vi "Start Stream.vi"(8 "error in (no error)":errorcluster, 10 "Camera Settings":T1={"Exposure Time (ms)"=100.0, "Binning"=enum."2x2", "Scan Mode"=0, "Frames to Acquire"=1000.0, "Pixel Correction"=FALSE, "Frames to Skip"=0, "File Path"=path "", "Duty cycle"=0.0, "ALEX"=FALSE, "Shutter Enable"=[], "Timelapse Interval (s)"=0, "fluidics trigger frame"=0} {"Timelapse Interval (s)" max=60000 step=1; "Exposure Time (ms)" min=1.0 max=10000.0 step=1.0}, 11 "Orca-Flash 4.0 V2 in":refnum<class "Hamamatsu Camera.lvclass">) -> (0 "error out":errorcluster, 3 "Orca-Flash 4.0 V2 out":refnum<class "Hamamatsu Camera.lvclass">)   [LabVIEW 2018, in "Hamamatsu Camera.lvlib" / "Hamamatsu Camera.lvclass"]
uses:
  Hamamatsu Camera.lvclass
  Resources/Type Defs/Camera Settings.ctl
  Camera/Camera.lvclass
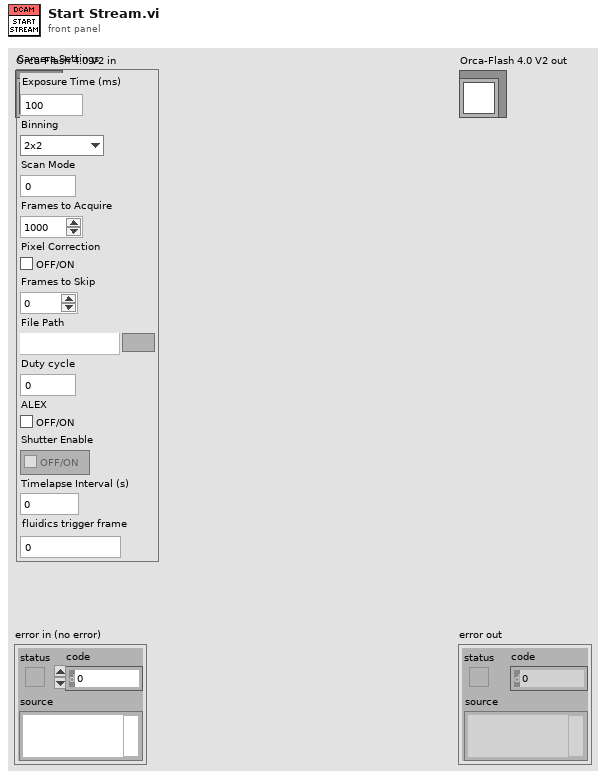
[diagram p1: front panel]
types:
  T1 = typedef "Camera Settings.ctl" = cluster{"Exposure Time (ms)":dbl, "Binning":enum16{"1x1", "2x2", "4x4"}, "Scan Mode":i32, "Frames to Acquire":dbl, "Pixel Correction":bool, "Frames to Skip":u32, "File Path":path, "Duty cycle":dbl, "ALEX":bool, "Shutter Enable":bool[], "Timelapse Interval (s)":u32, "fluidics trigger frame":u16}
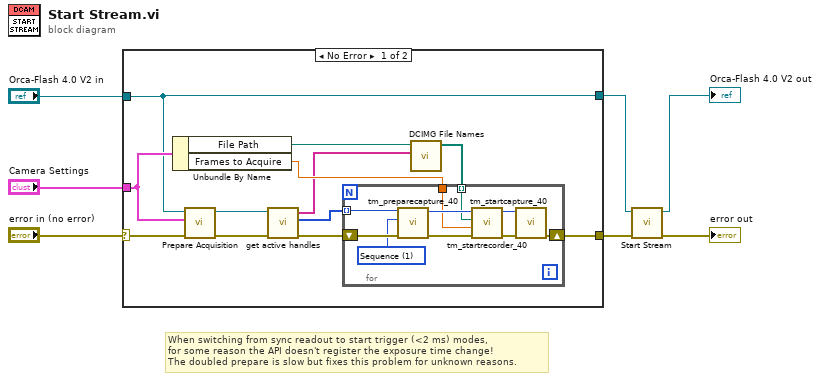
[diagram p0: block diagram]
diagram:
  # "When switching from sync readout to start trigger (<2 ms) modes,\nfor some reason the API doesn't register the exposure time change!\nThe doubled prepare is slow but fixes this problem for unknown reasons."
  n1 = case shown="No Error" "error in (no error)" {
    selector: "error in (no error)" -> [w16 w31]
    tunnel: [w8 w31] -> w3
    tunnel: [w9 w30] -> w2
    tunnel: "Orca-Flash 4.0 V2 in" -> [w9 w30]
    tunnel: "Camera Settings" -> [w17 _]
    frame No Error {
      n2 = Unbundle By Name(w17) -> ("File Path"=w18:path, "Frames to Acquire"=w15:dbl)
      n3 = call "Prepare Acquisition.vi"("error in (no error)"=w16, "Flash Settings"=w17, "Orca-Flash 4.0 in"=w9) -> ("error out"=w10:errorcluster, "Orca-Flash 4.0 out"=w11:refnum<class "Hamamatsu Camera.lvclass">)  [unwired: 7 in]
      n4 = call-dynamic "get active handles.vi"("error in (no error)"=w10, "Hamamatsu Camera in"=w11) -> ("error out"=w14:errorcluster, "Handles"=w13:u32[], "Camera Names"=w12:string[])  [unwired: 5 in, 2 out]
      n5 = call "DCIMG File Names.vi"("Channel Names"=w12, "TIFF File Path"=w18) -> ("DCIMG Files"=w19:path[])  [unwired: 9 in]
      n6 = for {
        tunnel: w13 -> [w24] mode=indexing
        shift-right: [w21] -> w8
        shift-left: w14 -> [w29]
        tunnel: w19 -> [w22] mode=indexing
        tunnel: w15 -> [w20]
        w23 = 1 items=["Snap", "Sequence"] ("Capture mode")
        n7 = call <userlib>:"tm_preparecapture_40.vi"("error in (no error)"=w29, "Capture mode"=w23, "Handle in"=w24) -> ("error out"=w28:errorcluster, "Handle out"=w25:u32)  [unwired: 5 in, 2 out]
        n8 = call <userlib>:"tm_startrecorder_40.vi"("error in (no error)"=w28, "frames"=w20, "File"=w22, "Handle in"=w25) -> ("error out"=w27:errorcluster, "Handle out"=w26:u32)  [unwired: 6 in]
        n9 = call <userlib>:"tm_startcapture_40.vi"("error in (no error)"=w27, "Handle in"=w26) -> ("error out"=w21:errorcluster)  [unwired: 8 in, 1 out]
      }
    }
    frame Error {
    }
  }
  n10 = call-parent "Start Stream.vi"("error in (no error)"=w3, "Camera in"=w2) -> ("error out"=→"error out":errorcluster, "Camera out"=→"Orca-Flash 4.0 V2 out":refnum<class "Hamamatsu Camera.lvclass">)  [unwired: 8 in]
